vi "Flush Endpoint.vi"(8 "error in (no error)":errorcluster, 11 "Stream in":refnum<class "Stream.lvclass">) -> (0 "error out":errorcluster, 3 "Stream out":refnum<class "Stream.lvclass">)   [LabVIEW 2018]
uses:
  Stream.lvclass
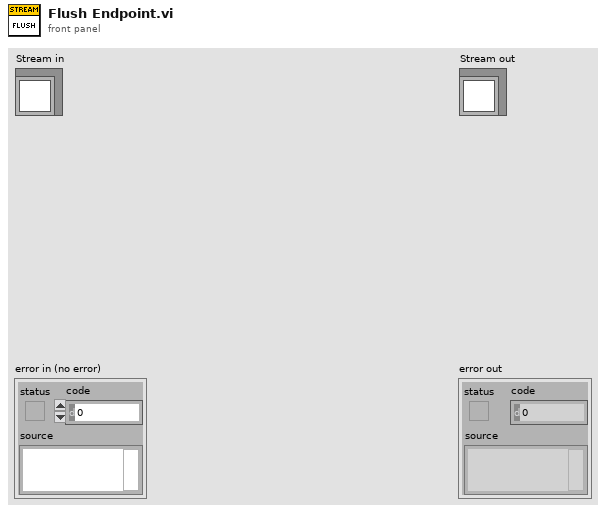
[diagram p1: front panel]
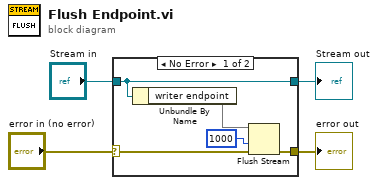
[diagram p0: block diagram]
diagram:
  n1 = case shown="No Error" "error in (no error)" {
    selector: "error in (no error)" -> [w8 w11]
    tunnel: [w9 w11] -> w3
    tunnel: [w6 w10] -> w1
    tunnel: "Stream in" -> [w6 w10]
    frame No Error {
      n2 = Unbundle By Name(w6) -> ("writer endpoint"=w5)
      n3 = Flush Stream(8:w8, 9:1000 ("timeout in ms (-1)"), 11:w5) -> (0:w9:errorcluster)  [unwired: 1 in, 2 out]
    }
    frame Error {
    }
  }
  "error out" <- w3
  "Stream out" <- w1
